vi "RT Main.vi"() -> ()   [LabVIEW 2013]
doc: "This template is for the Queued Message Handler design pattern.\n\nThe Event Handling Loop generates messages based on user interface actions.\n\nThe Message Handling Loop processes messages generated by the Event Handling Loop, or by other messages. The messages are string values, so new messages can be added easily to the Message Cases case structure in the Message Handling Loop. Each message cluster can also provide an optional value for Message Data, which is a variant that can be converted to whatever message-specific data is required."
uses:
  <vilib>/userdefined/High Color/nirio_resource_hc.ctl
  controls/FPGA State.ctl
  controls/Raw Values.ctl
  controls/Control Configuration.ctl
  controls/Custom Controller Inputs.ctl
  Globals/Global - All RT Loop Stop.vi
  Globals/Global - Configuration Options.vi
  <vilib>/rvi/errors/niLvFpgaAdjustHostInterfaceError.vi
  Globals/Global - RT Stream Connections.vi
  <vilib>/FPGAPlugInAG/cRIO-9075/niLvFpga_Close_cRIO-9075.vi
  <vilib>/rvi/interface/nirviReadWriteControl/nirviReadWriteControl.xnode
  controls/FPGA VI Reference.ctl
  FPGA Bitfiles/crio-FPGA-contro_FPGATarget_FPGAMain_4HKUk4gb9wY.lvbitx
  <vilib>/rvi/interface/nirviCloseFPGA/nirviCloseFPGA.xnode
  support/Message Queue/Message Queue.lvlib
  NiFpgaLv.dll
  <vilib>/nisyscfg/nisyscfg.lvlib
  <instrlib>/ZaberTSeries/ZaberTSeries.lvlib
panel:
  in  "VISA resource name":refnum<visa-resource-name>
  in  "cRIO resource name":T1
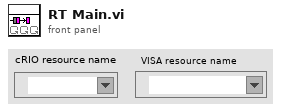
[diagram p1: front panel]
types:
  T1 = typedef "nirio_resource_hc.ctl" = tag
  T2 = typedef "FPGA VI Reference.ctl" = refnum<k20>
  T3 = typedef "FPGA State.ctl" = enum16{"Safe State", "Manual", "Control (PID)"}
  T4 = typedef "Control Configuration.ctl" = cluster{"PID Gains":cluster{"proportional gain (Kc)":fxp<+/-,16,8>, "integral gain (Kc*Ts/Ti)":fxp<+/-,16,8>, "derivative gain (Kc*Td/Ts)":fxp<+/-,16,8>}, "Output Range":cluster{"output high":fxp<+/-,16,7>, "output low":fxp<+/-,16,7>}}
  T5 = typedef "Custom Controller Inputs.ctl" = cluster{"Other Controller Gains":cluster{"kvc (N/m)":fxp<+,16,12>, "ymod (-)":fxp<+/-,16,5>, "Mar (kg)":fxp<+/-,16,8>, "bp (kg/s)":fxp<+/-,16,5>, "Foff (N)":fxp<+/-,16,8>, "Fthresh (N)":fxp<+/-,16,5>}}
  T6 = typedef "Raw Values.ctl" = cluster{"Channel 0":fxp<+/-,20,7>, "Channel 1":fxp<+/-,20,7>, "Channel 2":fxp<+/-,20,7>, "Channel 3":fxp<+/-,20,14>}
  T7 = typedef "All FPGA Configuration Values.ctl" = cluster{"FPGA State":T3, "Manual Values":T6, "Setpoints":T6, "Control Configurations":T4[]}
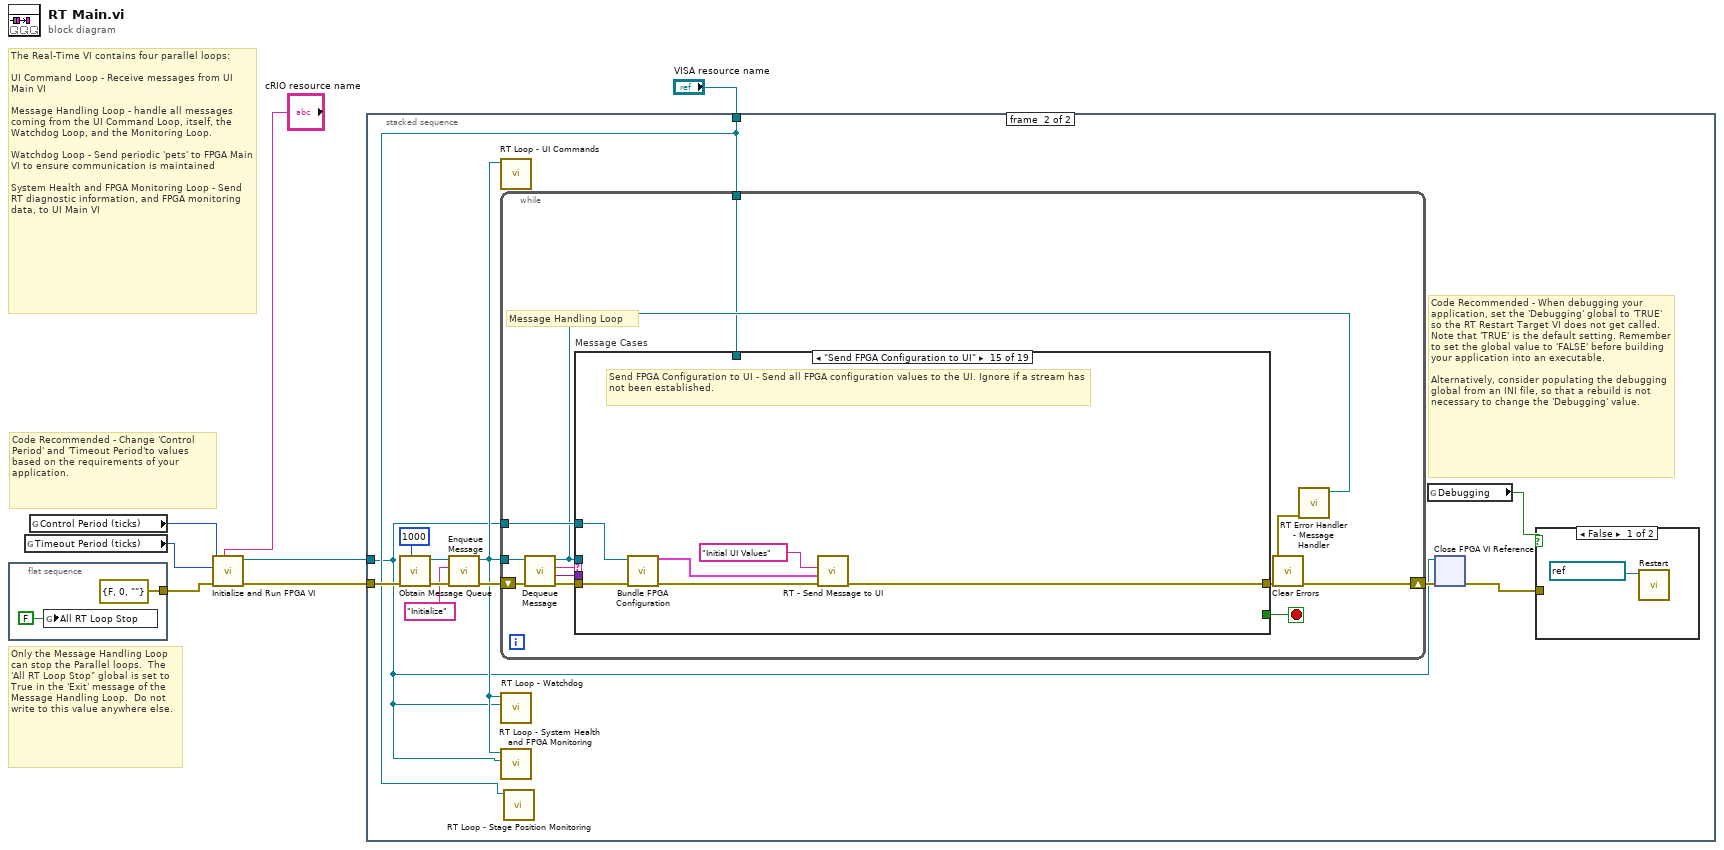
[diagram p0: block diagram]
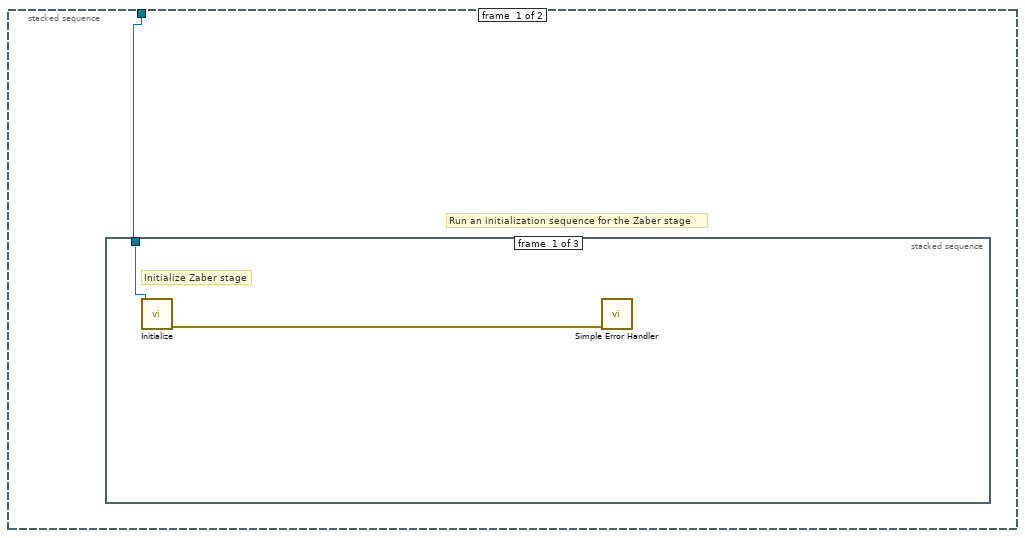
[diagram p2: hidden frame]
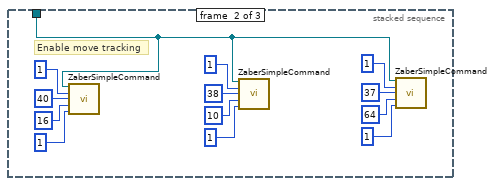
[diagram p3: hidden frame]
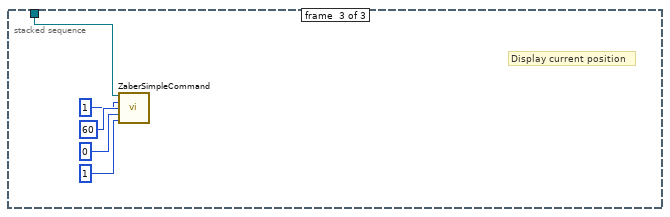
[diagram p4: hidden frame]
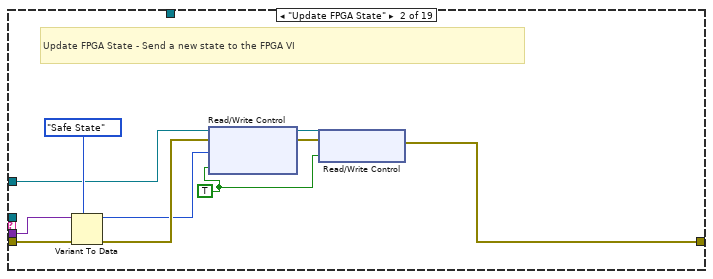
[diagram p7: hidden frame]
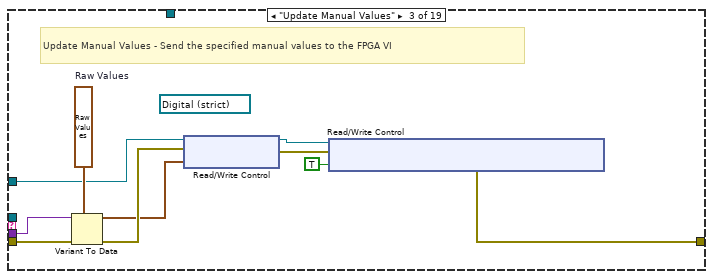
[diagram p8: hidden frame]
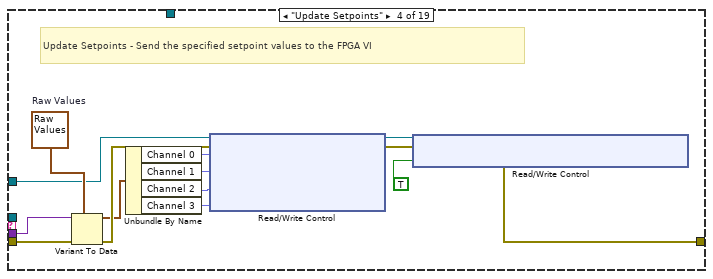
[diagram p9: hidden frame]
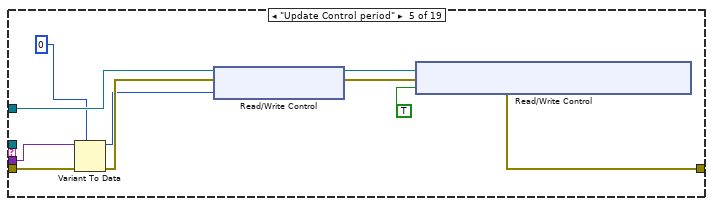
[diagram p10: hidden frame]
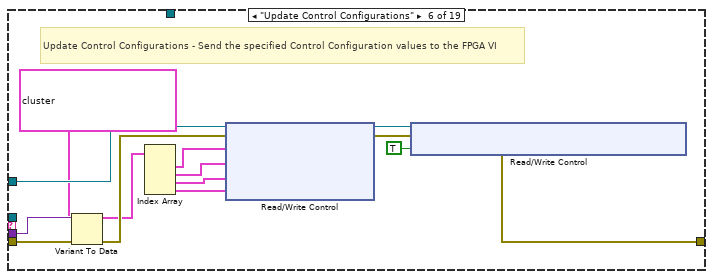
[diagram p11: hidden frame]
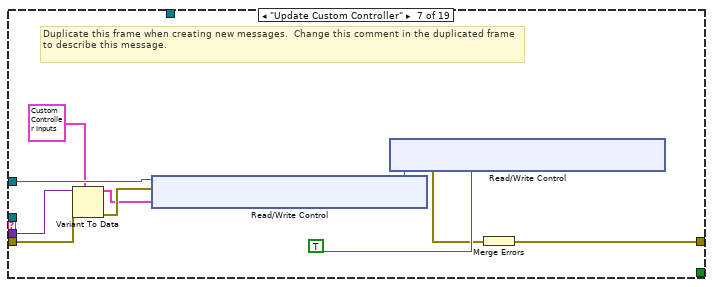
[diagram p12: hidden frame]
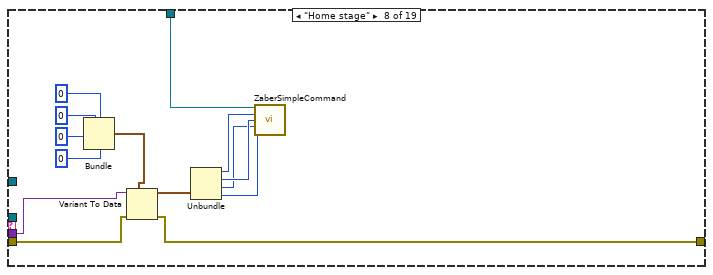
[diagram p13: hidden frame]
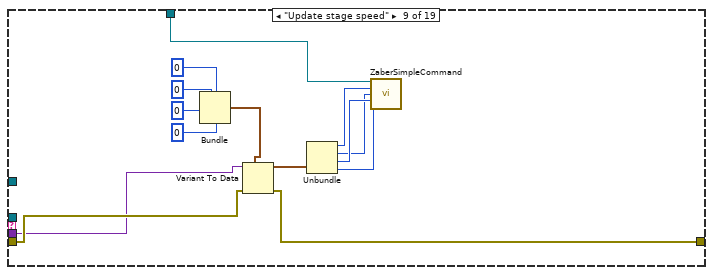
[diagram p14: hidden frame]
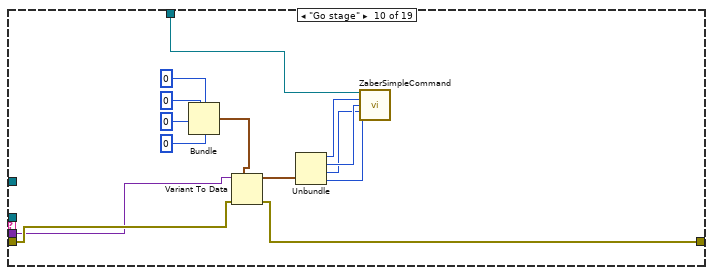
[diagram p15: hidden frame]
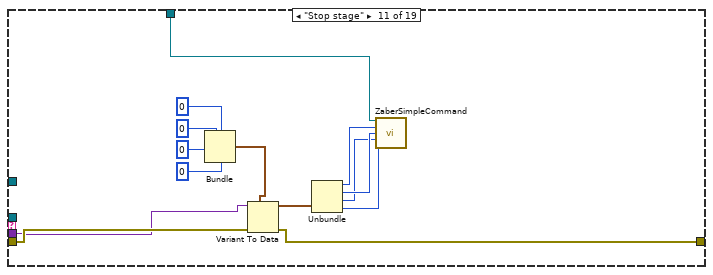
[diagram p16: hidden frame]
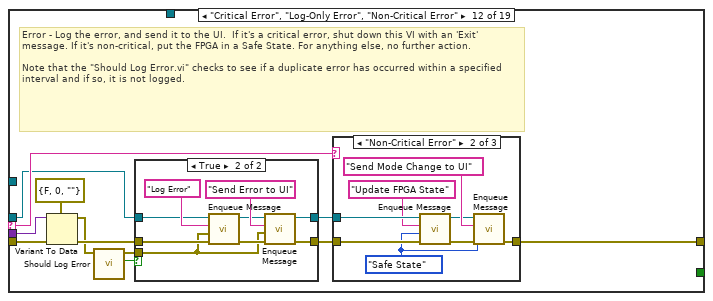
[diagram p17: hidden frame]
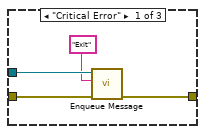
[diagram p19: hidden frame]
diagram:
  # "Code Recommended - Change 'Control Period' and 'Timeout Period'to values based on the requirements of your application."
  # "The Real-Time VI contains four parallel loops:\n\nUI Command Loop - Receive messages from UI Main VI\n\nMessage Handling Loop - handle all messages coming from the UI Command Loop, itself, the Watchdog Loop, and the Monitoring Loop.\n\nWatchdog Loop - Send periodic 'pets' to FPGA Main VI to ensure communication is maintained\n\nSystem Health and FPGA Monitoring Loop - Send RT diagnostic information, and FPGA monitoring data, to UI Main VI"
  # "Only the Message Handling Loop can stop the Parallel loops.  The 'All RT Loop Stop\" global is set to True in the 'Exit' message of the Message Handling Loop.  Do not write to this value anywhere else."
  n1 = flat-sequence {
    tunnel: [errorcluster {"status"=FALSE, "code"=0, "source"=""} ("error constant")] -> w6
    frame #0 {
      n2 = global write "Global - All RT Loop Stop.vi" "All RT Loop Stop"(FALSE) -> ()
    }
  }
  n3 = global read "Global - Configuration Options.vi" "Timeout Period (ticks)"() -> (w4:u64)
  n4 = global read "Global - Configuration Options.vi" "Control Period (ticks)"() -> (w5:u32)
  n5 = call "Initialize and Run FPGA VI.vi"("resource name"="cRIO resource name", "error in (no error)"=w6, "Timeout Period (ticks)"=w4, "Control Period (ticks)"=w5) -> ("error out"=w7:errorcluster, "FPGA VI Reference Out"=w3:T2)  [unwired: 6 in]
  n6 = stacked-sequence {
    tunnel: w7 -> [_ w33]
    tunnel: w3 -> [_ w31]
    tunnel: "VISA resource name" -> [w10 w32]
    frame #0 {
      # "Run an initialization sequence for the Zaber stage"
      n7 = stacked-sequence {
        tunnel: w10 -> [w11 w13 w26]
        frame #0 {
          # "Initialize Zaber stage"
          n8 = call <instrlib>:"Initialize.vi"("VISA resource name"=w11) -> ("error out"=w12:errorcluster)  [unwired: 8 in, 2 out]
          n9 = call <vilib>:"Simple Error Handler.vi"("error in (no error)"=w12) -> ()  [unwired: 4 in, 5 out]
        }
        frame #1 {
          # "Enable move tracking"
          n10 = call "ZaberSimpleCommand.vi"("VISA Refnum in"=w13, "Num1"=1, "Cmd"=40, "Val"=16, "Resp num"=1) -> ()  [unwired: 8 in, 3 out]
          n11 = call "ZaberSimpleCommand.vi"("VISA Refnum in"=w13, "Num1"=1, "Cmd"=38, "Val"=10, "Resp num"=1) -> ()  [unwired: 8 in, 3 out]
          n12 = call "ZaberSimpleCommand.vi"("VISA Refnum in"=w13, "Num1"=1, "Cmd"=37, "Val"=64, "Resp num"=1) -> ()  [unwired: 8 in, 3 out]
        }
        frame #2 {
          # "Display current position"
          n13 = call "ZaberSimpleCommand.vi"("VISA Refnum in"=w26, "Num1"=1, "Cmd"=60, "Val"=0, "Resp num"=1) -> ()  [unwired: 8 in, 3 out]
        }
      }
    }
    frame #1 {
      # "Code Recommended - When debugging your application, set the 'Debugging' global to 'TRUE' so the RT Restart Target VI does not get called.  Note that 'TRUE' is the default setting. Remember to set the global value to 'FALSE' before building your application into an executable.\n\nAlternatively, consider populating the debugging global from an INI file, so that a rebuild is not necessary to change the 'Debugging' value."
      n14 = call "Obtain Message Queue.vi"("max queue size (-1, unlimited)"=1000, "error in (no error)"=w33) -> ("error out"=w42:errorcluster, "Message Queue"=w41:refnum<queue>)  [unwired: 8 in]
      n15 = call "Enqueue Message.vi"("error in (no error)"=w42, "Message"="Initialize", "Message Queue"=w41) -> ("error out"=w39:errorcluster, "dup Message Queue"=w38:refnum<queue>)  [unwired: 7 in]
      n16 = call "RT Loop - UI Commands.vi"("Message Queue"=w38) -> ()  [unwired: 11 in]
      n17 = while {
        tunnel: w38 -> [w49]
        shift-right: [w46] -> w37
        shift-left: w39 -> [w53]
        tunnel: w31 -> [w48]
        tunnel: w32 -> [w44]
        stop <- w54 stop-if-true
        # "Message Handling Loop"
        n18 = call "Dequeue Message.vi"("error in (no error)"=w53, "Message Queue"=w49) -> ("error out"=w52:errorcluster, "Message Data"=w50:variant, "Message"=w51:string, "dup Message Queue"=w47:refnum<queue>)  [unwired: 6 in]
        n19 = case "Message Cases" shown="\"Send FPGA Configuration to UI\"" w51 {
          selector: w51 -> [_ _ _ _ _ _ _ _ _ _ _ w190 _ _ _ _ _ _ w261]
          tunnel: w47 -> [_ _ _ _ _ _ _ _ _ _ _ w184 _ _ _ _ w255 _ _]
          tunnel: w52 -> [w55 w65 w75 w89 w94 w113 w123 w137 w142 w156 w170 w188 w227 w231 w237 w241 w251 w257 _]
          tunnel: [w55 w57 w66 w76 w95 w100 w124 w136 w139 w153 w169 w189 w218 w228 w232 w240 w252 w256 w259] -> w45
          tunnel: [_ _ _ _ _ _ _ _ _ _ _ _ _ _ _ _ TRUE _ _] -> w54
          tunnel: w50 -> [_ w64 w74 w88 w93 w112 w122 w135 w141 w155 w168 w187 w226 w230 _ w239 _ _ _]
          tunnel: w48 -> [_ w61 w71 w85 w92 w110 w121 _ _ _ _ _ _ _ w236 _ w247 _ _]
          tunnel: w44 -> [_ _ _ _ _ _ _ w138 w140 w154 w167 _ _ _ _ _ _ _ _]
          frame "Initialize" {
            # "Initialize - Currently a no-op for the RT Main VI"
          }
          frame "Update FPGA State" {
            w56 = TRUE ("Change State")
            # "Update FPGA State - Send a new state to the FPGA VI"
            n20 = Variant To Data(error in=w65, type=FPGA_State."Safe State" ("FPGA State"), Variant=w64) -> (data=w60:T3, error out=w62:errorcluster)
            n21 = xnode "Read/Write Control"("FPGA VI Reference In"=w61, "error in"=w62, "New State"=w60, "Change State"=w56) -> ("FPGA VI Reference Out"=w59:T2, "error out"=w58:errorcluster)
            n22 = xnode "Read/Write Control"("FPGA VI Reference In"=w59, "error in"=w58, "Disable Drive"=w56) -> ("error out"=w57:errorcluster)  [unwired: 1 out]
          }
          frame "Update Manual Values" {
            (unwired) refnum<vi> refnum ("Control period (ticks) Ref")
            w73 = T6 {"Channel 0"=0.0, "Channel 1"=0.0, "Channel 2"=0.0, "Channel 3"=0.0}  # Raw Values
            # "Update Manual Values - Send the specified manual values to the FPGA VI"
            n23 = Variant To Data(error in=w75, type=w73, Variant=w74) -> (data=w70:T6, error out=w72:errorcluster)
            n24 = xnode "Read/Write Control"("FPGA VI Reference In"=w71, "error in"=w72, "Manual Values"=w70) -> ("FPGA VI Reference Out"=w69:T2, "error out"=w68:errorcluster)
            n25 = xnode "Read/Write Control"("FPGA VI Reference In"=w69, "error in"=w68, "Enable Drive"=TRUE) -> ("error out"=w66:errorcluster)  [unwired: 1 out]
          }
          frame "Update Setpoints" {
            w87 = T6 {"Channel 0"=0.0, "Channel 1"=0.0, "Channel 2"=0.0, "Channel 3"=0.0}  # Raw Values
            # "Update Setpoints - Send the specified setpoint values to the FPGA VI"
            n26 = Variant To Data(error in=w89, type=w87, Variant=w88) -> (data=w84:T6, error out=w86:errorcluster)
            n27 = Unbundle By Name(w84) -> ("Channel 0"=w83:fxp<+/-,20,7>, "Channel 1"=w80:fxp<+/-,20,7>, "Channel 2"=w82:fxp<+/-,20,7>, "Channel 3"=w81:fxp<+/-,20,14>)
            n28 = xnode "Read/Write Control"("FPGA VI Reference In"=w85, "error in"=w86, "Channel 0 Setpoint (Force)"=w83, "Channel 1 Setpoint  (Position)"=w80, "Channel 2 Setpoint"=w82, "Channel 3 Setpoint"=w81) -> ("FPGA VI Reference Out"=w77:T2, "error out"=w78:errorcluster)
            n29 = xnode "Read/Write Control"("FPGA VI Reference In"=w77, "error in"=w78, "Enable Drive"=TRUE) -> ("error out"=w76:errorcluster)  [unwired: 1 out]
          }
          frame "Update Control period" {
            n30 = Variant To Data(error in=w94, type=u32 0 ("Control period (ticks)"), Variant=w93) -> (data=w90:u32, error out=w96:errorcluster)
            n31 = xnode "Read/Write Control"("FPGA VI Reference In"=w92, "error in"=w96, "Control Period (ticks)"=w90) -> ("FPGA VI Reference Out"=w99:T2, "error out"=w98:errorcluster)
            n32 = xnode "Read/Write Control"("FPGA VI Reference In"=w99, "error in"=w98, "Enable Drive"=TRUE) -> ("error out"=w95:errorcluster)  [unwired: 1 out]
          }
          frame "Update Control Configurations" {
            # "Update Control Configurations - Send the specified Control Configuration values to the FPGA VI"
            n33 = Variant To Data(error in=w113, type=T4[] [{"PID Gains"={"proportional gain (Kc)"=0.0, "integral gain (Kc*Ts/Ti)"=0.0, "derivative gain (Kc*Td/Ts)"=0.0}, "Output Range"={"output high"=0.0, "output low"=0.0}}], Variant=w112) -> (data=w108:T4[], error out=w111:errorcluster)
            n34 = Index Array(array=w108) -> (element #1=w107:T4, element #2=w106:T4, element #3=w105:T4, element #4=w104:T4)  [unwired: 4 in]
            n35 = xnode "Read/Write Control"("FPGA VI Reference In"=w110, "error in"=w111, "Channel 0 Configuration"=w107, "Channel 1 Configuration"=w106, "Channel 2 Configuration"=w105, "Channel 3 Configuration"=w104) -> ("FPGA VI Reference Out"=w102:T2, "error out"=w101:errorcluster)
            n36 = xnode "Read/Write Control"("FPGA VI Reference In"=w102, "error in"=w101, "Enable Drive"=TRUE) -> ("error out"=w100:errorcluster)  [unwired: 1 out]
          }
          frame "Update Custom Controller" {
            # "Duplicate this frame when creating new messages.  Change this comment in the duplicated frame to describe this message."
            n37 = Variant To Data(error in=w123, type=T5 {"Other Controller Gains"={"kvc (N/m)"=0.0, "ymod (-)"=0.0, "Mar (kg)"=0.0, "bp (kg/s)"=0.0, "Foff (N)"=0.0, "Fthresh (N)"=0.0}} ("Custom Controller Inputs"), Variant=w122) -> (data=w115:T5, error out=w120:errorcluster)
            n38 = xnode "Read/Write Control"("FPGA VI Reference In"=w121, "error in"=w120, "Custom Controller Inputs"=w115) -> ("FPGA VI Reference Out"=w118:T2, "error out"=w117:errorcluster)
            n39 = xnode "Read/Write Control"("FPGA VI Reference In"=w118, "error in"=w117, "Enable Drive"=TRUE) -> ("error out"=w116:errorcluster)  [unwired: 1 out]
            n40 = Merge Errors(w116) -> (w124:errorcluster)
          }
          frame "Home stage" {
            n41 = Bundle(0, 0, 0, 0) -> (w130:cluster{i32, i32, i32, i32})  [unwired: 1 in]
            n42 = Variant To Data(error in=w137, type=w130, Variant=w135) -> (data=w129:cluster{i32, i32, i32, i32}, error out=w136:errorcluster)
            n43 = Unbundle(w129) -> (w128:i32, w127:i32, w126:i32, w125:i32)
            n44 = call "ZaberSimpleCommand.vi"("VISA Refnum in"=w138, "Num1"=w128, "Cmd"=w127, "Val"=w126, "Resp num"=w125) -> ()  [unwired: 8 in, 3 out]
          }
          frame "Update stage speed" {
            n45 = Bundle(0, 0, 0, 0) -> (w147:cluster{i32, i32, i32, i32})  [unwired: 1 in]
            n46 = Variant To Data(error in=w142, type=w147, Variant=w141) -> (data=w148:cluster{i32, i32, i32, i32}, error out=w139:errorcluster)
            n47 = Unbundle(w148) -> (w149:i32, w150:i32, w151:i32, w152:i32)
            n48 = call "ZaberSimpleCommand.vi"("VISA Refnum in"=w140, "Num1"=w149, "Cmd"=w150, "Val"=w151, "Resp num"=w152) -> ()  [unwired: 8 in, 3 out]
          }
          frame "Go stage" {
            n49 = Bundle(0, 0, 0, 0) -> (w162:cluster{i32, i32, i32, i32})  [unwired: 1 in]
            n50 = Variant To Data(error in=w156, type=w162, Variant=w155) -> (data=w161:cluster{i32, i32, i32, i32}, error out=w153:errorcluster)
            n51 = Unbundle(w161) -> (w160:i32, w159:i32, w158:i32, w157:i32)
            n52 = call "ZaberSimpleCommand.vi"("VISA Refnum in"=w154, "Num1"=w160, "Cmd"=w159, "Val"=w158, "Resp num"=w157) -> ()  [unwired: 8 in, 3 out]
          }
          frame "Stop stage" {
            n53 = Bundle(0, 0, 0, 0) -> (w176:cluster{i32, i32, i32, i32})  [unwired: 1 in]
            n54 = Variant To Data(error in=w170, type=w176, Variant=w168) -> (data=w175:cluster{i32, i32, i32, i32}, error out=w169:errorcluster)
            n55 = Unbundle(w175) -> (w174:i32, w173:i32, w172:i32, w171:i32)
            n56 = call "ZaberSimpleCommand.vi"("VISA Refnum in"=w167, "Num1"=w174, "Cmd"=w173, "Val"=w172, "Resp num"=w171) -> ()  [unwired: 8 in, 3 out]
          }
          frame "Critical Error", "Log-Only Error", "Non-Critical Error" {
            # "Error - Log the error, and send it to the UI.  If it's a critical error, shut down this VI with an 'Exit' message. If it's non-critical, put the FPGA in a Safe State. For anything else, no further action.\n\nNote that the \"Should Log Error.vi\" checks to see if a duplicate error has occurred within a specified interval and if so, it is not logged."
            n57 = Variant To Data(error in=w188, type=errorcluster {"status"=FALSE, "code"=0, "source"=""} ("error out"), Variant=w187) -> (data=w182:errorcluster, error out=w185:errorcluster)
            n58 = call "Should Log Error.vi"("error to report"=w182) -> ("Should Log Error?"=w183:bool, "dup error to report"=w181:errorcluster)  [unwired: 9 in]
            n59 = case shown="True" w183 {
              tunnel: [w194 w201] -> w192
              tunnel: [w193 w200] -> w191
              tunnel: w184 -> [w193 w199]
              tunnel: w185 -> [w194 w196]
              tunnel: w181 -> [_ w195]
              frame False {
              }
              frame True {
                n60 = call "Enqueue Message.vi"("error in (no error)"=w196, "Message Data"=w195, "Message"="Log Error", "Message Queue"=w199) -> ("error out"=w197:errorcluster, "dup Message Queue"=w198:refnum<queue>)  [unwired: 6 in]
                n61 = call "Enqueue Message.vi"("error in (no error)"=w197, "Message Data"=w195, "Message"="Send Error to UI", "Message Queue"=w198) -> ("error out"=w201:errorcluster, "dup Message Queue"=w200:refnum<queue>)  [unwired: 6 in]
              }
            }
            n62 = case shown="\"Non-Critical Error\"" w190 {
              tunnel: w192 -> [w207 w215 w216]
              tunnel: w191 -> [w205 w214 _]
              tunnel: [w206 w211 w216] -> w189
              frame "Critical Error" {
                n63 = call "Enqueue Message.vi"("error in (no error)"=w207, "Message"="Exit", "Message Queue"=w205) -> ("error out"=w206:errorcluster)  [unwired: 7 in, 1 out]
              }
              frame "Non-Critical Error" {
                w208 = FPGA_State."Safe State" ("FPGA State")
                n64 = call "Enqueue Message.vi"("error in (no error)"=w215, "Message Data"=w208, "Message"="Update FPGA State", "Message Queue"=w214) -> ("error out"=w212:errorcluster, "dup Message Queue"=w209:refnum<queue>)  [unwired: 6 in]
                n65 = call "Enqueue Message.vi"("error in (no error)"=w212, "Message Data"=w208, "Message"="Send Mode Change to UI", "Message Queue"=w209) -> ("error out"=w211:errorcluster)  [unwired: 6 in, 1 out]
              }
              frame Default {
              }
            }
          }
          frame "Log Error" {
            # "Log Error - Log the error, along with a timestamp, to the RT log file."
            n66 = Variant To Data(error in=w227, type=errorcluster {"status"=FALSE, "code"=0, "source"=""} ("error constant"), Variant=w226) -> (data=w221:errorcluster, error out=w224:errorcluster)
            n67 = Unbundle By Name(w221) -> ("code"=w220:i32, "source"=w219:string)
            n68 = Format Date/Time String() -> (date/time string=w222:string)  [unwired: 3 in]
            n69 = Format Into String(format string="\n%s: RT Error %d - %s", w222, w220, w219) -> (resulting string=w217:string)  [unwired: 2 in, 1 out]
            n70 = call "Write to RT Error Log.vi"("error in (no error)"=w224, "Log Entry"=w217) -> ("error out"=w218:errorcluster)  [unwired: 9 in]
          }
          frame "Send Error to UI" {
            # "Send Error to UI - Send the error message to the UI. Ignore if a stream has not been established."
            n71 = call "RT - Send Message to UI.vi"("error in (no error)"=w231, "Message Data"=w230, "Message"="RT Error") -> ("error out"=w228:errorcluster)  [unwired: 8 in]
          }
          frame "Send FPGA Configuration to UI" {
            # "Send FPGA Configuration to UI - Send all FPGA configuration values to the UI. Ignore if a stream has not been established."
            n72 = call "Bundle FPGA Configuration.vi"("error in (no error)"=w237, "FPGA Interface (Old)"=w236) -> ("error out"=w235:errorcluster, "All FPGA Configuration Values"=w234:T7)  [unwired: 8 in]
            n73 = call "RT - Send Message to UI.vi"("error in (no error)"=w235, "Message Data"=w234, "Message"="Initial UI Values") -> ("error out"=w232:errorcluster)  [unwired: 8 in]
          }
          frame "Send Mode Change to UI" {
            # "Send Mode Change to UI - Let the UI Main VI know that the mode of the FPGA Main VI has changed."
            n74 = call "RT - Send Message to UI.vi"("error in (no error)"=w241, "Message Data"=w239, "Message"="Update Display Mode") -> ("error out"=w240:errorcluster)  [unwired: 8 in]
          }
          frame "Exit" {
            # "Flush the Writer Stream to ensure all pending messages are sent to UI Main VI"
            # "Destroy streams on exit"
            # "Put FPGA VI in a Safe State on Exit"
            # "Stop Message Handling Loop"
            # "Stop All Parallel Loops"
            # "Release the message queue reference"
            n75 = global read "Global - RT Stream Connections.vi" "RT Writer Stream"() -> (w244:refnum<k21>)
            n76 = global read "Global - RT Stream Connections.vi" "UI Writer Stream"() -> (w246:refnum<k21>)
            n77 = Flush Stream(11:w244) -> (0:w242:errorcluster, 3:w243:refnum<k21>)  [unwired: 3 in, 1 out]
            n78 = Release Queue(queue=w255, error in (no error)=w251) -> (error out=w253:errorcluster)  [unwired: 1 in, 2 out]
            n79 = Destroy Stream Endpoint(8:w242, 11:w243) -> (0:w245:errorcluster)
            n80 = Destroy Stream Endpoint(8:w245, 11:w246) -> ()  [unwired: 1 out]
            n81 = xnode "Read/Write Control"("FPGA VI Reference In"=w247, "New State"=FPGA_State."Safe State", "Change State"=TRUE) -> ()  [unwired: 1 in, 2 out]
            n82 = global write "Global - All RT Loop Stop.vi" "All RT Loop Stop"(TRUE ("Stop Monitoring Loops")) -> ()
            n83 = Merge Errors(w253) -> (w252:errorcluster)
          }
          frame "---Copy This Frame---" {
            # "Duplicate this frame when creating new messages.  Change this comment in the duplicated frame to describe this message."
            n84 = Merge Errors(w257) -> (w256:errorcluster)
          }
          frame Default {
            # "'Default' case only runs if there is a message that isn't defined in any of the other cases.  Output a programming error."
            n85 = Format Into String(format string="The invalid message string \"%s\" was received in the Message Handling Loop." ("Unknown Message Error Text"), w261) -> (resulting string=w258:string)  [unwired: 2 in, 1 out]
            n86 = call <vilib>:"Error Cluster From Error Code.vi"("error message (\"\")"=w258, "error code (0)"=1) -> ("error out"=w259:errorcluster)  [unwired: 7 in]
          }
        }
        n87 = call <vilib>:"Clear Errors.vi"("error in (no error)"=w45) -> ("error out"=w46:errorcluster)  [unwired: 6 in]
        n88 = call "RT Error Handler - Message Handler.vi"("error in (no error)"=w45, "Message Queue"=w47) -> ()  [unwired: 9 in, 1 out]
      }
      n89 = call "RT Loop - Watchdog.vi"("FPGA VI Reference Out"=w31, "Message Queue"=w38) -> ()  [unwired: 10 in]
      n90 = call "RT Loop - System Health and FPGA Monitoring.vi"("FPGA VI Reference Out"=w31, "Message Queue"=w38) -> ()  [unwired: 10 in]
      n91 = call "RT Loop - Stage Position Monitoring.vi"("VISA resource name"=w32) -> ()  [unwired: 11 in]
      n92 = global read "Global - Configuration Options.vi" "Debugging"() -> (w35:bool)
      n93 = xnode "Close FPGA VI Reference"("FPGA VI Reference In"=w31, "error in"=w37) -> ("error out"=w36:errorcluster)
      n94 = case shown="False" w35 {
        tunnel: w36 -> [_ _]
        frame False {
          n95 = call <vilib>:"Restart.vi"("session in"=refnum<k21> "localhost") -> ()  [unwired: 8 in, 3 out]
        }
        frame True {
        }
      }
    }
  }
